vi "Current VI's Path (VI or exe).vi"() -> (6 "Full Path to VI or executable":path, 10 "VI or executable installation directory":path)   [LabVIEW 2017]
doc: "Current VI's Path (VI or exe).vi\n\n<B>Description:</B>\n\nThe Current VI's Path (VI or exe) VI is a drop-in replacement for the native Current VI's Path function. Just replace the native Current VI's Path function in your application with the Current VI's Path (VI or exe) VI and you'll never have to deal with the frustration caused by bad paths again -- whether you run your code in the development environment or as an executable!\n\nThe Current VI's Path (VI or exe) VI gets the path to the VI that called it and searches that path for \".exe\". If \".exe\" is found in the path, then the Current VI's Path (VI or exe) VI strips the path twice to obtain the executable's installation directory. If \".exe\" is not found, then the Current VI's Path (VI or exe) VI strips the path once to obtain the VI's installation directory.\n\nIn either case, the Current VI's Path (VI or exe) VI returns the VI or executable installation directory and the Full Path to the VI or executable. You can use this information in your application to easily access sub folders of the VI's or executable's installation directory by using the Build Path function to append the sub directory's name to the VI's or executable's installation path returned by the Current VI's Path (VI or exe) VI.\n\n<B>Usage:</B>\n\nUse the Current VI's Path (VI or exe) VI wherever you would use the native Current VI's Path function.\n\n<B>NOTES:</B>\n\nNone.\n\n<B>Inputs:</B>\n\nNone.\n\n<B>Outputs:</B>\n\nFull Path to VI or executable - The full path to the VI or executable.\n\nVI or executable installation directory - The path to the installation directory of the VI or executable.\n\n<B>Developed by:</B>\n\nMark Ridgley\nMark.Ridgley_LabVIEW.Developer@comcast.net"
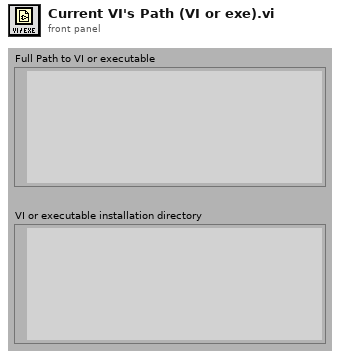
[diagram p1: front panel]
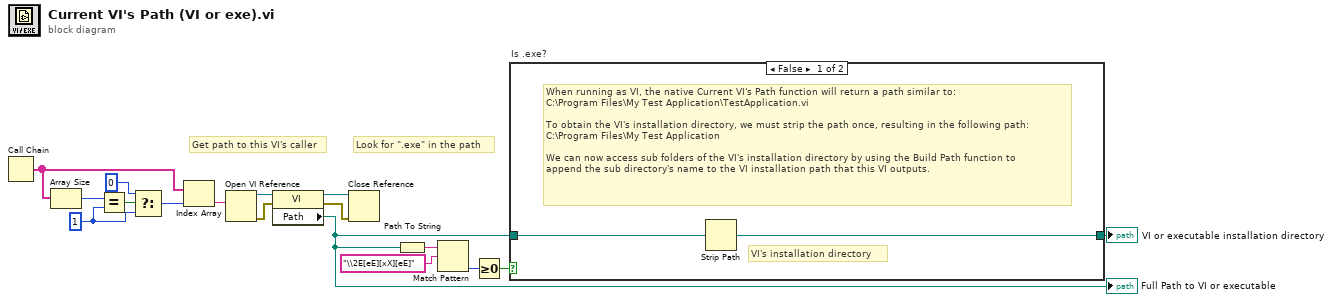
[diagram p0: block diagram]
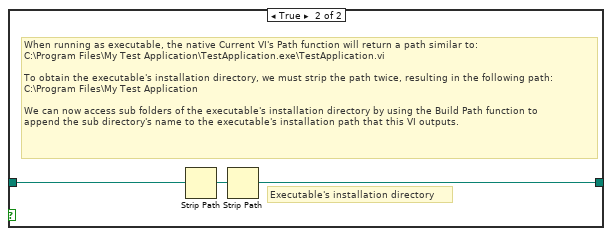
[diagram p2: hidden frame]
diagram:
  w8 = 1 ("index")
  # "Get path to this VI's caller"
  # "Look for \".exe\" in the path"
  n1 = Call Chain() -> (call chain=w12:string[])
  n2 = Array Size(array=w12) -> (size(s)=w9:i32)
  n3 = Equal?(x=w9, y=w8) -> (x = y?=w11:bool)
  n4 = Select(t=0, s=w11, f=w8) -> (s? t:f=w10:i32)
  n5 = Index Array(array=w12, index=w10) -> (element=w4:string)
  n6 = Open VI Reference(vi path=w4) -> (vi reference=w5:refnum<vi>, error out=w6:errorcluster)  [unwired: 5 in]
  n7 = property class="VI"(reference=w5, error in=w6) -> (reference out=w1:refnum<vi>, error out=w2:errorcluster, "Path"=w3:path)
  "Full Path to VI or executable" <- w3
  n8 = Close Reference(reference=w1, error in (no error)=w2) -> ()  [unwired: 1 out]
  n9 = Path To String(path=w3) -> (string=w14:string)
  n10 = Match Pattern(string=w14, regular expression="\\2E[eE][xX][eE]") -> (offset past match=w16:i32)  [unwired: 1 in, 3 out]
  n11 = Greater Or Equal To 0?(x=w16) -> (x >= 0?=w15:bool)
  n12 = case "Is .exe?" shown="False" w15 {
    tunnel: w3 -> [w19 w22]
    tunnel: [w18 w20] -> w17
    frame False {
      # "VI's installation directory"
      # "When running as VI, the native Current VI's Path function will return a path similar to:\nC:\\Program Files\\My Test Application\\TestApplication.vi\n\nTo obtain the VI's installation directory, we must strip the path once, resulting in the following path:\nC:\\Program Files\\My Test Application\n\nWe can now access sub folders of the VI's installation directory by using the Build Path function to\nappend the sub directory's name to the VI installation path that this VI outputs."
      n13 = Strip Path(path=w19) -> (stripped path=w18:path)  [unwired: 1 out]
    }
    frame True {
      # "Executable's installation directory"
      # "When running as executable, the native Current VI's Path function will return a path similar to:\nC:\\Program Files\\My Test Application\\TestApplication.exe\\TestApplication.vi\n\nTo obtain the executable's installation directory, we must strip the path twice, resulting in the following path:\nC:\\Program Files\\My Test Application\n\nWe can now access sub folders of the executable's installation directory by using the Build Path function to\nappend the sub directory's name to the executable's installation path that this VI outputs."
      n14 = Strip Path(path=w22) -> (stripped path=w21:path)  [unwired: 1 out]
      n15 = Strip Path(path=w21) -> (stripped path=w20:path)  [unwired: 1 out]
    }
  }
  "VI or executable installation directory" <- w17
